vi "Graph_Arrow.vi"() -> ()   [LabVIEW 2009]
panel:
  out "Heading 2":dbl
  out "cos(x)":dbl
  out "sin(x)":dbl
  in  "magnitude":dbl
  in  "Heading":dbl step=15.0
  out "XY Graph":T1(graph)
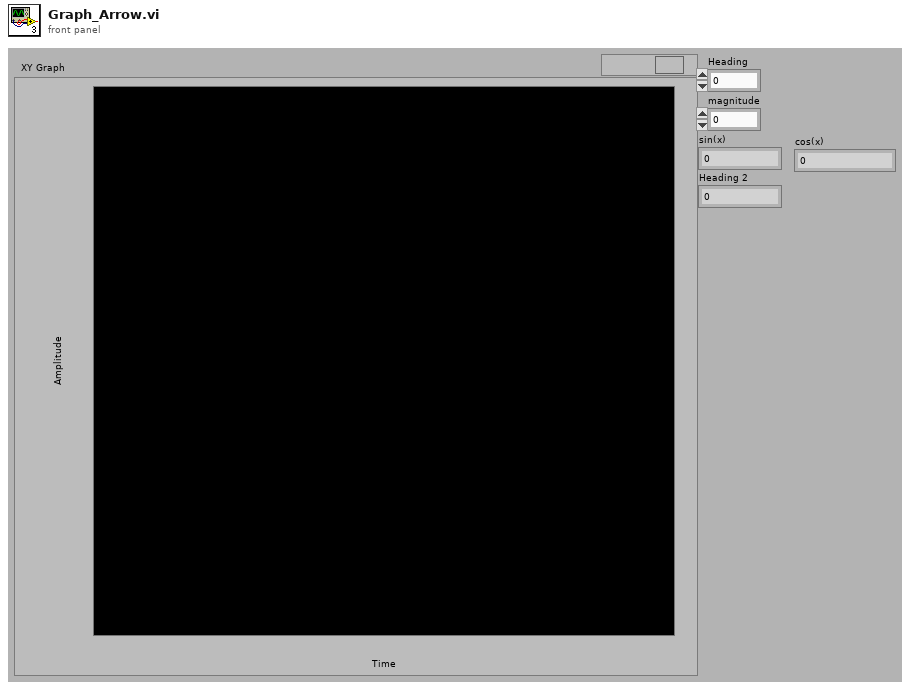
[diagram p1: front panel]
types:
  T1 = cluster{"initialized array":dbl[], "initialized array":dbl[]}[]
  T2 = cluster{"initialized array":dbl[], "initialized array":dbl[]}
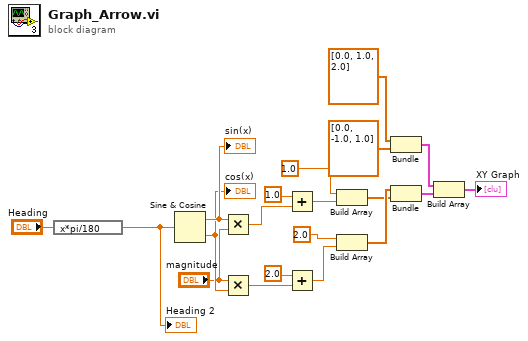
[diagram p0: block diagram]
diagram:
  n1 = expression code="x*pi/180"("Heading") -> (w15:dbl)
  "Heading 2" <- w15
  n2 = Sine & Cosine(0:w15) -> (1:w14:dbl, 2:w13:dbl)
  "sin(x)" <- w14
  "cos(x)" <- w13
  n3 = Multiply(x=w14, y="magnitude") -> (x*y=w4:dbl)
  n4 = Multiply(x="magnitude", y=w13) -> (x*y=w6:dbl)
  n5 = Add(x=1.0, y=w4) -> (x+y=w3:dbl)
  n6 = Add(x=2.0, y=w6) -> (x+y=w5:dbl)
  n7 = Build Array(1.0 ("x"), w3) -> (w10:dbl[])
  n8 = Build Array(2.0 ("x"), w5) -> (w11:dbl[])
  n9 = Bundle("initialized array"=dbl[] [0.0, 1.0, 2.0], "initialized array"=dbl[] [0.0, -1.0, 1.0]) -> (w18:T2)  [unwired: 1 in]
  n10 = Bundle(w11, w10) -> (w9:cluster{dbl[], dbl[]})  [unwired: 1 in]
  n11 = Build Array(w18, w9) -> (→"XY Graph":T1)
